vi "svl_Decimate Resampled Level Signal (N Ch).vi"(6 "actual time constant [rev]":dbl format="%.2f", 7 "decimation factor":i32, 8 "error in (no error)":errorcluster, 9 "processing state":T1(ring), 11 "scaled signals":T2(array[cluster]) {"even angle signal" format="%.2f"; "dr" format="%.2f"; "r0" format="%.2f"}) -> (0 "error out":errorcluster, 3 "decimated signals":T2(array[cluster]) {"even angle signal" format="%.2f"; "dr" format="%.2f"; "r0" format="%.2f"}, 4 "dup actual time constant [rev]":dbl format="%.2f", 5 "actual decimation factor":i32)   [LabVIEW 2017]
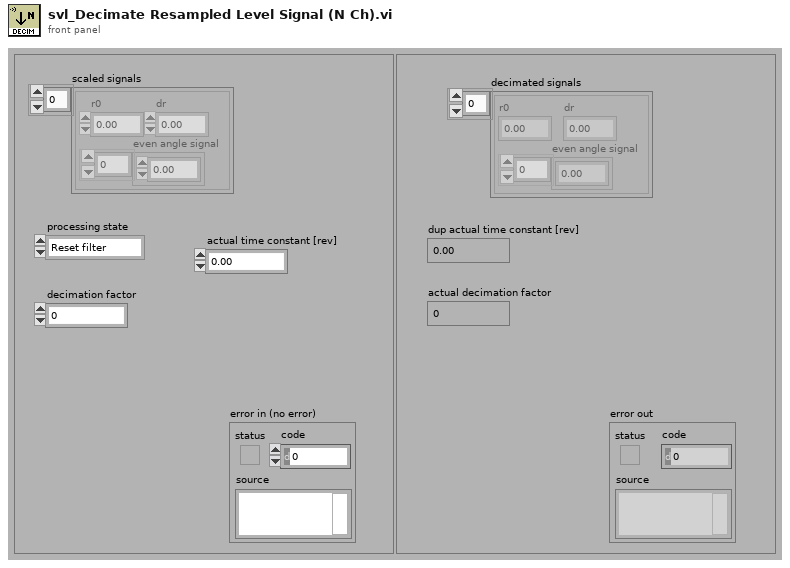
[diagram p1: front panel]
types:
  T1 = enum16{"Reset filter", "Restart averaging", "Continue processing"}
  T2 = cluster{"r0":dbl, "dr":dbl, "even angle signal":dbl[]}[]
  T3 = cluster{"r0":dbl, "dr":dbl, "even angle signal":dbl[]}
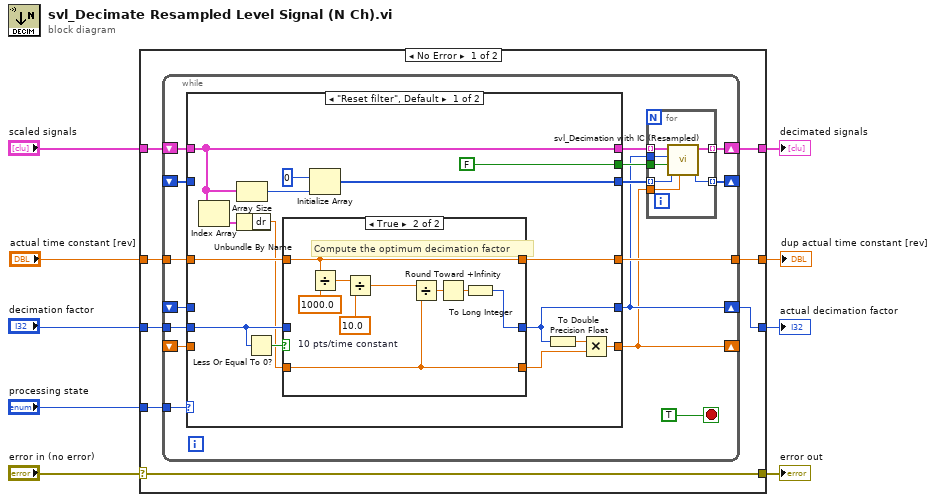
[diagram p0: block diagram]
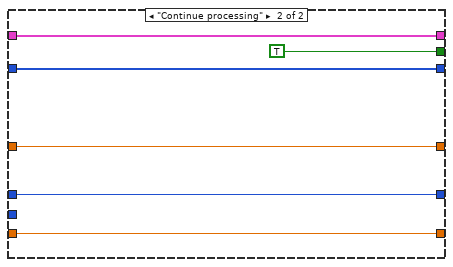
[diagram p3: hidden frame]
diagram:
  n1 = case shown="No Error" "error in (no error)" {
    selector: "error in (no error)" -> [w16 w77]
    tunnel: [w16 w77] -> w8
    tunnel: "actual time constant [rev]" -> [w17 w75]
    tunnel: "processing state" -> [w15 _]
    tunnel: "scaled signals" -> [w14 w76]
    tunnel: "decimation factor" -> [w10 w74]
    tunnel: [w12 w76] -> w3
    tunnel: [w13 w75] -> w2
    tunnel: [w11 w74] -> w1
    frame No Error {
      n2 = while {
        shift-left: _ -> [w28]
        shift-right: [w24] -> _
        tunnel: [w30] -> w13
        tunnel: w15 -> [w32]
        tunnel: w17 -> [w33]
        shift-right: [w18] -> _
        shift-left: _ -> [w22]
        shift-right: [w19] -> w11
        shift-left: _ -> [w20]
        tunnel: w10 -> [w21]
        shift-right: [w23] -> w12
        shift-left: w14 -> [w31]
        stop <- TRUE stop-if-true
        n3 = case shown="\"Reset filter\", Default" w32 {
          tunnel: w31 -> [w43 w71]
          tunnel: [w43 w71] -> w27
          tunnel: [w44 w70] -> w26
          tunnel: w33 -> [w54 w73]
          tunnel: [w48 w69] -> w19
          tunnel: w21 -> [w52 _]
          tunnel: [w53 w73] -> w30
          tunnel: [w46 w68] -> w18
          tunnel: w28 -> [_ w70]
          tunnel: [FALSE ("init/cont (init:F)") TRUE ("init/cont (init:F)")] -> w25
          tunnel: w22 -> [_ w68]
          tunnel: w20 -> [_ w69]
          frame "Reset filter", Default {
            n4 = Index Array(array=w43) -> (element=w42:T3)  [unwired: 1 in]
            n5 = Array Size(array=w43) -> (size(s)=w45:i32)
            n6 = Unbundle By Name(w42) -> ("dr"=w41:dbl)
            n7 = Less Or Equal To 0?(x=w52) -> (x <= 0?=w55:bool)
            n8 = case shown="True" w55 {
              tunnel: [w56 w59] -> w47
              tunnel: [w57 w61] -> w48
              tunnel: w54 -> [w58 w60]
              tunnel: [w58 w60] -> w53
              tunnel: w41 -> [w56 w59]
              tunnel: w52 -> [w57 _]
              frame False {
                # "User defined decimation factor"
              }
              frame True {
                w67 = 10.0  # 10 pts/time constant
                # "Compute the optimum decimation factor"
                n9 = Divide(x=w60, y=1000.0) -> (x/y=w64:dbl)
                n10 = Divide(x=w64, y=w67) -> (x/y=w66:dbl)
                n11 = Divide(x=w66, y=w59) -> (x/y=w63:dbl)
                n12 = Round Toward +Infinity(x=w63) -> (ceil(x): smallest int >= x=w62:dbl)
                n13 = To Long Integer(number=w62) -> (32bit integer=w61:i32)
              }
            }
            n14 = Initialize Array(0 ("final decimation state"), w45) -> (w44:i32[])
            n15 = To Double Precision Float(number=w48) -> (double precision float=w49:dbl)
            n16 = Multiply(x=w49, y=w47) -> (x*y=w46:dbl)
          }
          frame "Continue processing" {
          }
        }
        n17 = for {
          tunnel: w27 -> [w40] mode=indexing
          tunnel: w26 -> [w39] mode=indexing
          tunnel: [w38] -> w23 mode=indexing
          tunnel: [w37] -> w24 mode=indexing
          tunnel: w19 -> [w36]
          tunnel: w25 -> [w35]
          tunnel: w18 -> [w34]
          n18 = call <vilib>:"svl_Decimation with IC (Resampled).vi"("new dr"=w34, "initial decimation state"=w39, "init/cont (init:F)"=w35, "decimating factor (1)"=w36, "even angle signal"=w40) -> ("final decimation state"=w37:i32, "even angle signal"=w38:T3)  [unwired: 5 in]
        }
      }
    }
    frame Error {
    }
  }
  "dup actual time constant [rev]" <- w2
  "decimated signals" <- w3
  "error out" <- w8
  "actual decimation factor" <- w1
